vi "benchmark-tagContainer.vi"() -> (3 "write":dbl[](array[numeric])=[4.609181880950928e-05, 2.400779724121094e-06, 7.494449615478516e-07, 2.3156785964965823e-05, 0.00027759432792663576] caption="average" format="%#_6p")   [LabVIEW 2017]
uses:
  c133460f-0aec-4b14-aa01-684956f011bf.vi
  679e9543-87f0-4a91-8f0b-568c5a8b50fd.vi
  TagDB/_Support/DataAccess/_NameCacher.vi
  TagDB/_Support/DataAccess/_datatypeChecker.vi
  TagDB/_Support/DataAccess/TagDB Ref to DVR.vi
  <vilib>/Utility/Data Type/Get Type Information.vi
  <vilib>/Utility/error.llb/Trim Whitespace.vi
  TagDB/_Support/Error/_[error50000]Invalid DB REF.vi
  TagDB/_Support/Error/_[error50002]Invalid DataType.vi
  TagDB/TagDB(DEV).lvlib
panel:
  out "error out":errorcluster
  in  "group name in (Untitled)":string="add more data to containerprivate data"
  out "length":i32=1170
  out "unit (ms)":cluster{dbl[]}[](graph)=[{[4.501104354858398e-05, 5.501508712768555e-05, 6.0143470764160154e-05, 4.501104354858398e-05, 4.500865936279297e-05, 4.001379013061524e-05, 4.5013427734375e-05, 4.000663757324219e-05, 4.500865936279297e-05, 4.5013427734375e-05, 4.5013427734375e-05, 4.5006275177001956e-05, 4.500865936279297e-05, 6.0017108917236326e-05, 4.5123100280761717e-05, 4.500865936279297e-05, 4.500865936279297e-05, 4.5015811920166016e-05, 4.5013427734375e-05, 4.5015811920166016e-05, 4.501104354858398e-05, 4.500865936279297e-05, 5.010128021240234e-05, 4.500865936279297e-05, 4.501104354858398e-05, 4.5013427734375e-05, 4.5006275177001956e-05, 4.500865936279297e-05, 4.501104354858398e-05, 4.502296447753906e-05, 4.5013427734375e-05, 4.500865936279297e-05, 4.501104354858398e-05, 4.501104354858398e-05, 4.5013427734375e-05, 5.0008296966552734e-05, 6.501436233520508e-05, 4.5013427734375e-05, 4.5006275177001956e-05, 4.5013427734375e-05, 4.500865936279297e-05, 4.501104354858398e-05, 5.001068115234375e-05, 4.5013427734375e-05, 4.500865936279297e-05, 4.501104354858398e-05, 4.500865936279297e-05, 4.500865936279297e-05, 4.5013427734375e-05, 4.5013427734375e-05, 4.5006275177001956e-05, 4.500865936279297e-05, 5.001544952392578e-05, 4.500865936279297e-05, 4.501104354858398e-05, 5.501508712768555e-05, 4.5015811920166016e-05, 4.500865936279297e-05, 4.253387451171875e-05, 4.501104354858398e-05, 4.500865936279297e-05, 4.500865936279297e-05, 4.501104354858398e-05, 4.5003890991210935e-05, 4.502058029174805e-05, 4.5015811920166016e-05, 4.5003890991210935e-05, 4.5013427734375e-05, 4.501104354858398e-05, 4.7619342803955076e-05, 4.753589630126953e-05, 4.501104354858398e-05, 4.500865936279297e-05, 5.254030227661133e-05, 4.500865936279297e-05, 4.5006275177001956e-05, 4.5013427734375e-05, 4.500865936279297e-05, 5.000591278076172e-05, 5.001544952392578e-05, 5.003213882446289e-05, 4.5015811920166016e-05, 4.5013427734375e-05, 4.501104354858398e-05, 4.5015811920166016e-05, 4.500865936279297e-05, 4.500865936279297e-05, 4.500865936279297e-05, 4.500865936279297e-05, 4.500865936279297e-05, 4.500865936279297e-05, 4.501104354858398e-05, 4.500865936279297e-05, 4.502296447753906e-05, 4.7540664672851564e-05, 4.501104354858398e-05, 4.5013427734375e-05, 4.501104354858398e-05, 4.500865936279297e-05, 4.500865936279297e-05]}, {[0.0, 0.0, 0.0, 4.999637603759765e-06, 0.0, 4.999637603759765e-06, 4.999637603759765e-06, 5.0044059753417965e-06, 0.0, 4.999637603759765e-06, 0.0, 5.002021789550781e-06, 4.999637603759765e-06, 0.0, 0.0, 0.0, 4.999637603759765e-06, 5.002021789550781e-06, 5.002021789550781e-06, 0.0, 5.002021789550781e-06, 5.0044059753417965e-06, 0.0, 0.0, 0.0, 0.0, 0.0, 4.999637603759765e-06, 4.999637603759765e-06, 5.0044059753417965e-06, 0.0, 0.0, 5.002021789550781e-06, 0.0, 0.0, 0.0, 0.0, 5.002021789550781e-06, 5.0044059753417965e-06, 4.999637603759765e-06, 0.0, 0.0, 0.0, 5.002021789550781e-06, 0.0, 5.002021789550781e-06, 5.0091743469238285e-06, 0.0, 0.0, 4.999637603759765e-06, 4.999637603759765e-06, 4.999637603759765e-06, 0.0, 5.0044059753417965e-06, 5.0044059753417965e-06, 4.999637603759765e-06, 4.99725341796875e-06, 5.002021789550781e-06, 5.0044059753417965e-06, 0.0, 5.0044059753417965e-06, 0.0, 4.999637603759765e-06, 0.0, 0.0, 0.0, 0.0, 0.0, 4.999637603759765e-06, 0.0, 0.0, 4.999637603759765e-06, 5.0044059753417965e-06, 5.0044059753417965e-06, 4.999637603759765e-06, 0.0, 4.999637603759765e-06, 0.0, 0.0, 0.0, 0.0, 0.0, 0.0, 0.0, 4.99725341796875e-06, 0.0, 0.0, 5.002021789550781e-06, 0.0, 5.0067901611328125e-06, 0.0, 5.0044059753417965e-06, 5.0044059753417965e-06, 5.002021789550781e-06, 0.0, 4.999637603759765e-06, 4.999637603759765e-06, 0.0, 4.999637603759765e-06, 0.0]}, {[4.999637603759765e-06, 0.0, 4.963874816894531e-06, 0.0, 0.0, 0.0, 0.0, 0.0, 0.0, 0.0, 4.999637603759765e-06, 0.0, 0.0, 0.0, 4.9686431884765625e-06, 0.0, 0.0, 0.0, 0.0, 4.994869232177734e-06, 0.0, 0.0, 0.0, 0.0, 0.0, 5.0044059753417965e-06, 5.0044059753417965e-06, 0.0, 0.0, 0.0, 0.0, 0.0, 0.0, 0.0, 0.0, 0.0, 0.0, 0.0, 0.0, 0.0, 5.0044059753417965e-06, 0.0, 0.0, 0.0, 0.0, 0.0, 0.0, 0.0, 0.0, 0.0, 0.0, 0.0, 0.0, 0.0, 0.0, 0.0, 0.0, 0.0, 0.0, 0.0, 0.0, 4.999637603759765e-06, 0.0, 0.0, 0.0, 0.0, 0.0, 4.999637603759765e-06, 0.0, 0.0, 0.0, 0.0, 0.0, 0.0, 0.0, 0.0, 0.0, 0.0, 0.0, 0.0, 0.0, 4.99725341796875e-06, 0.0, 0.0, 0.0, 4.999637603759765e-06, 5.0044059753417965e-06, 0.0, 5.0044059753417965e-06, 0.0, 0.0, 0.0, 0.0, 0.0, 0.0, 0.0, 0.0, 4.999637603759765e-06, 0.0, 0.0]}, {[0.0, 4.999637603759765e-06, 0.0, 0.0, 5.0044059753417965e-06, 5.0044059753417965e-06, 4.999637603759765e-06, 5.0044059753417965e-06, 5.002021789550781e-06, 5.0044059753417965e-06, 4.999637603759765e-06, 4.999637603759765e-06, 5.0044059753417965e-06, 9.99927520751953e-06, 5.0044059753417965e-06, 1.0008811950683593e-05, 1.0004043579101563e-05, 1.0004043579101563e-05, 1.0004043579101563e-05, 5.002021789550781e-06, 1.0004043579101563e-05, 9.99927520751953e-06, 1.5003681182861328e-05, 1.5003681182861328e-05, 1.5001296997070313e-05, 9.9945068359375e-06, 9.99927520751953e-06, 9.99927520751953e-06, 1.0001659393310548e-05, 1.4998912811279296e-05, 1.4998912811279296e-05, 1.5003681182861328e-05, 1.5003681182861328e-05, 1.5003681182861328e-05, 2.0003318786621095e-05, 1.500844955444336e-05, 2.000570297241211e-05, 1.5020370483398438e-05, 1.4996528625488281e-05, 2.0003318786621095e-05, 1.4998912811279296e-05, 2.0008087158203125e-05, 2.0003318786621095e-05, 2.0000934600830078e-05, 2.0003318786621095e-05, 2.0008087158203125e-05, 1.999855041503906e-05, 2.0008087158203125e-05, 2.500295639038086e-05, 2.500772476196289e-05, 2.5010108947753908e-05, 2.500772476196289e-05, 2.5005340576171874e-05, 2.5019645690917968e-05, 2.5000572204589844e-05, 2.500772476196289e-05, 2.500295639038086e-05, 2.5005340576171874e-05, 2.5005340576171874e-05, 3.0007362365722656e-05, 2.500295639038086e-05, 2.5019645690917968e-05, 3.0009746551513673e-05, 3.0009746551513673e-05, 3.0007362365722656e-05, 3.000020980834961e-05, 3.0007362365722656e-05, 3.0007362365722656e-05, 3.000497817993164e-05, 3.000497817993164e-05, 3.500938415527344e-05, 3.000497817993164e-05, 3.0007362365722656e-05, 3.5006999969482425e-05, 3.5016536712646485e-05, 4.001379013061524e-05, 3.501176834106445e-05, 3.5006999969482425e-05, 3.500938415527344e-05, 3.500938415527344e-05, 4.000663757324219e-05, 3.5006999969482425e-05, 4.0018558502197264e-05, 4.001140594482422e-05, 4.000663757324219e-05, 3.500938415527344e-05, 3.5006999969482425e-05, 4.00853157043457e-05, 4.000663757324219e-05, 4.0001869201660157e-05, 4.5013427734375e-05, 4.000663757324219e-05, 4.501104354858398e-05, 4.501104354858398e-05, 4.5013427734375e-05, 4.500865936279297e-05, 4.50277328491211e-05, 4.0009021759033204e-05, 4.502296447753906e-05, 4.500865936279297e-05]}, {[4.99725341796875e-06, 1.5001296997070313e-05, 1.5001296997070313e-05, 2.500772476196289e-05, 3.0014514923095703e-05, 3.0002593994140626e-05, 4.0009021759033204e-05, 7.001161575317382e-05, 5.0008296966552734e-05, 5.501031875610351e-05, 6.0017108917236326e-05, 6.501436233520508e-05, 9.001970291137695e-05, 7.501602172851562e-05, 8.501529693603515e-05, 8.502721786499023e-05, 9.001493453979492e-05, 9.501457214355468e-05, 0.00010502099990844727, 0.00011002302169799805, 0.00011460304260253906, 0.00012002706527709961, 0.00012503862380981446, 0.00013002872467041016, 0.00013503074645996094, 0.00014003753662109375, 0.00014503717422485353, 0.00015503644943237304, 0.00015503644943237304, 0.00016003608703613281, 0.00017004013061523439, 0.00017503976821899413, 0.0001806044578552246, 0.00019005537033081054, 0.00019505500793457031, 0.000200045108795166, 0.000200042724609375, 0.0002050495147705078, 0.00021507501602172852, 0.00021257638931274414, 0.0002850651741027832, 0.000225064754486084, 0.00023006439208984376, 0.0002350640296936035, 0.00025005578994750975, 0.00025007009506225583, 0.0002551603317260742, 0.0002612662315368652, 0.0002650594711303711, 0.0002700614929199219, 0.00031507015228271484, 0.0002850604057312012, 0.0002850627899169922, 0.00029006481170654294, 0.0003100800514221191, 0.00030506372451782226, 0.0003050851821899414, 0.0003100967407226563, 0.00032007217407226563, 0.0003250718116760254, 0.00033008813858032227, 0.0003400731086730957, 0.00034508228302001956, 0.00036509513854980467, 0.000355076789855957, 0.00035508394241333006, 0.000360107421875, 0.0003650808334350586, 0.0003751087188720703, 0.000380094051361084, 0.0003900885581970215, 0.0003901028633117676, 0.0004000997543334961, 0.000400092601776123, 0.00040830373764038085, 0.000417630672454834, 0.00041509151458740234, 0.0004601216316223145, 0.00046011924743652346, 0.00043509244918823244, 0.00044509649276733396, 0.00045510292053222654, 0.00046511411666870115, 0.00047010421752929687, 0.0004651880264282227, 0.0004701137542724609, 0.0004752612113952637, 0.0004801154136657715, 0.00048010826110839844, 0.0004943060874938965, 0.0004851078987121582, 0.0004952120780944825, 0.0005151128768920898, 0.0005301427841186523, 0.0005151152610778809, 0.0005151271820068359, 0.0005251169204711914, 0.00053358793258667, 0.0005626559257507324, 0.0005377078056335449]}]
  out "outside":i32=99
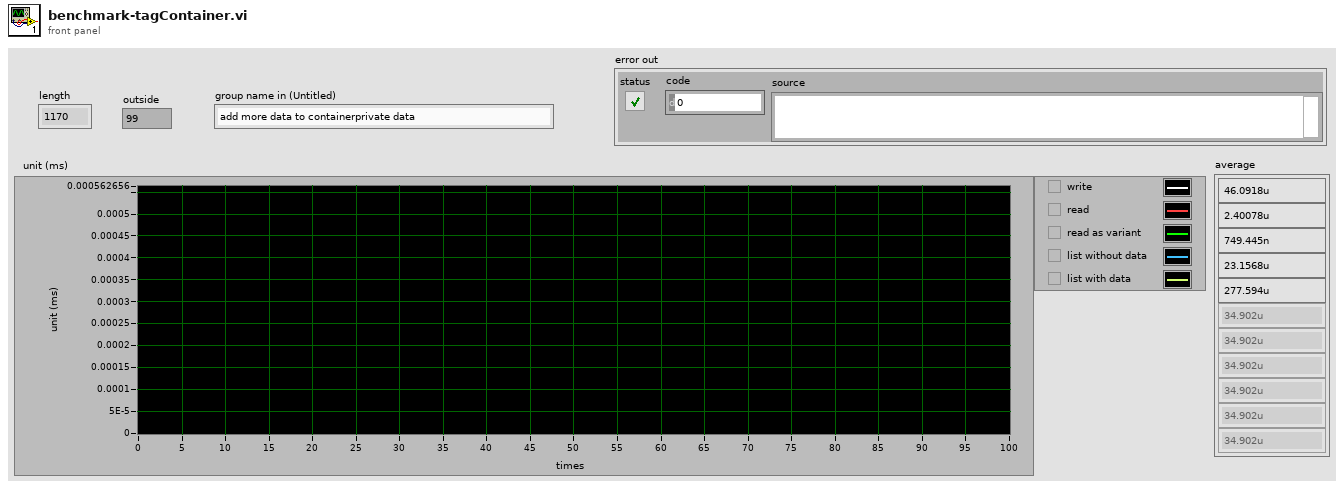
[diagram p1: front panel]
types:
  T1 = enum16{"open", "open or create", "create or replace", "create", "open (read-only)"}
  T2 = cluster{"error constant":errorcluster, "error constant 2":errorcluster, "error constant 3":errorcluster, "error constant 4":errorcluster, "error constant 5":errorcluster, "error constant 6":errorcluster, "error constant 7":errorcluster, "error constant 8":errorcluster, "error constant 9":errorcluster, "error constant 10":errorcluster, "error constant 11":errorcluster, "error constant 12":errorcluster, "error constant 13":errorcluster, "error constant 14":errorcluster, "error constant 15":errorcluster, "error constant 16":errorcluster, "error constant 17":errorcluster, "error constant 18":errorcluster, "error constant 19":errorcluster, "error constant 20":errorcluster, "error constant 21":errorcluster, "error constant 22":errorcluster, "error constant 23":errorcluster, "error constant 24":errorcluster, "error constant 25":errorcluster, "error constant 26":errorcluster, "error constant 27":errorcluster, "error constant 28":errorcluster, "error constant 29":errorcluster, "error constant 30":errorcluster, "error constant 31":errorcluster, "error constant 32":errorcluster, "error constant 33":errorcluster, "error constant 34":errorcluster, "error constant 35":errorcluster, "error constant 36":errorcluster, "error constant 37":errorcluster, "error constant 38":errorcluster, "error constant 39":errorcluster, "error constant 40":errorcluster, "error constant 41":errorcluster, "error constant 42":errorcluster, "error constant 43":errorcluster, "error constant 44":errorcluster, "error constant 45":errorcluster, "error constant 46":errorcluster, "error constant 47":errorcluster, "error constant 48":errorcluster, "error constant 49":errorcluster, "error constant 50":errorcluster, "error constant 51":errorcluster, "error constant 52":errorcluster, "error constant 53":errorcluster, "error constant 54":errorcluster, "error constant 55":errorcluster, "error constant 56":errorcluster, "error constant 57":errorcluster, "error constant 58":errorcluster, "error constant 59":errorcluster, "error constant 60":errorcluster, "error constant 61":errorcluster, "error constant 62":errorcluster, "error constant 63":errorcluster, "error constant 64":errorcluster, "error constant 65":errorcluster, cluster{"error constant":errorcluster, "error constant 2":errorcluster, "error constant 3":errorcluster, "error constant 4":errorcluster, "error constant 5":errorcluster, "error constant 6":errorcluster, "error constant 7":errorcluster, "error constant 8":errorcluster, "error constant 9":errorcluster, "error constant 10":errorcluster, "error constant 11":errorcluster, "error constant 12":errorcluster, "error constant 13":errorcluster, "error constant 14":errorcluster, "error constant 15":errorcluster, "error constant 16":errorcluster, "error constant 17":errorcluster, "error constant 18":errorcluster, "error constant 19":errorcluster, "error constant 20":errorcluster, "error constant 21":errorcluster, "error constant 22":errorcluster, "error constant 23":errorcluster, "error constant 24":errorcluster, "error constant 25":errorcluster, "error constant 26":errorcluster, "error constant 27":errorcluster, "error constant 28":errorcluster, "error constant 29":errorcluster, "error constant 30":errorcluster, "error constant 31":errorcluster, "error constant 32":errorcluster, "error constant 33":errorcluster, "error constant 34":errorcluster, "error constant 35":errorcluster, "error constant 36":errorcluster, "error constant 37":errorcluster, "error constant 38":errorcluster, "error constant 39":errorcluster, "error constant 40":errorcluster, "error constant 41":errorcluster, "error constant 42":errorcluster, "error constant 43":errorcluster, "error constant 44":errorcluster, "error constant 45":errorcluster, "error constant 46":errorcluster, "error constant 47":errorcluster, "error constant 48":errorcluster, "error constant 49":errorcluster, "error constant 50":errorcluster, "error constant 51":errorcluster, "error constant 52":errorcluster, "error constant 53":errorcluster, "error constant 54":errorcluster, "error constant 55":errorcluster, "error constant 56":errorcluster, "error constant 57":errorcluster, "error constant 58":errorcluster, "error constant 59":errorcluster, "error constant 60":errorcluster, "error constant 61":errorcluster, "error constant 62":errorcluster, "error constant 63":errorcluster, "error constant 64":errorcluster, "error constant 65":errorcluster}}
  T3 = typedef "TagDB(DEV).lvlib/TagContainer.ctl" = refnum<k1>
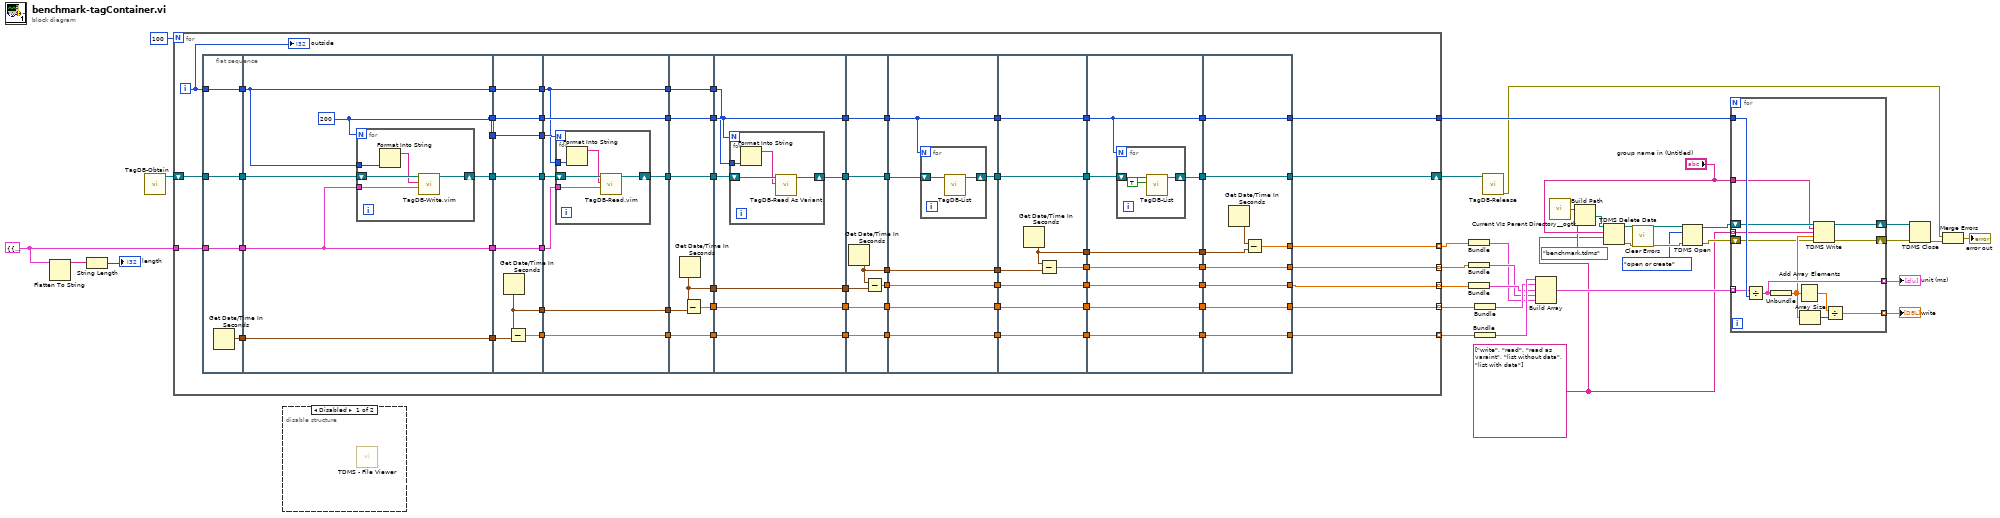
[diagram p0: block diagram]
diagram:
  w1 = string[] ["write", "read", "read as varaint", "list without data", "list with data"]
  w32 = T2 {"error constant"={"status"=FALSE, "code"=0, "source"=""}, "error constant 2"={"status"=FALSE, "code"=0, "source"=""}, "error constant 3"={"status"=FALSE, "code"=0, "source"=""}, "error constant 4"={"status"=FALSE, "code"=0, "source"=""}, "error constant 5"={"status"=FALSE, "code"=0, "source"=""}, "error constant 6"={"status"=FALSE, "code"=0, "source"=""}, "error constant 7"={"status"=FALSE, "code"=0, "source"=""}, "error constant 8"={"status"=FALSE, "code"=0, "source"=""}, "error constant 9"={"status"=FALSE, "code"=0, "source"=""}, "error constant 10"={"status"=FALSE, "code"=0, "source"=""}, "error constant 11"={"status"=FALSE, "code"=0, "source"=""}, "error constant 12"={"status"=FALSE, "code"=0, "source"=""}, "error constant 13"={"status"=FALSE, "code"=0, "source"=""}, "error constant 14"={"status"=FALSE, "code"=0, "source"=""}, "error constant 15"={"status"=FALSE, "code"=0, "source"=""}, "error constant 16"={"status"=FALSE, "code"=0, "source"=""}, "error constant 17"={"status"=FALSE, "code"=0, "source"=""}, "error constant 18"={"status"=FALSE, "code"=0, "source"=""}, "error constant 19"={"status"=FALSE, "code"=0, "source"=""}, "error constant 20"={"status"=FALSE, "code"=0, "source"=""}, "error constant 21"={"status"=FALSE, "code"=0, "source"=""}, "error constant 22"={"status"=FALSE, "code"=0, "source"=""}, "error constant 23"={"status"=FALSE, "code"=0, "source"=""}, "error constant 24"={"status"=FALSE, "code"=0, "source"=""}, "error constant 25"={"status"=FALSE, "code"=0, "source"=""}, "error constant 26"={"status"=FALSE, "code"=0, "source"=""}, "error constant 27"={"status"=FALSE, "code"=0, "source"=""}, "error constant 28"={"status"=FALSE, "code"=0, "source"=""}, "error constant 29"={"status"=FALSE, "code"=0, "source"=""}, "error constant 30"={"status"=FALSE, "code"=0, "source"=""}, "error constant 31"={"status"=FALSE, "code"=0, "source"=""}, "error constant 32"={"status"=FALSE, "code"=0, "source"=""}, "error constant 33"={"status"=FALSE, "code"=0, "source"=""}, "error constant 34"={"status"=FALSE, "code"=0, "source"=""}, "error constant 35"={"status"=FALSE, "code"=0, "source"=""}, "error constant 36"={"status"=FALSE, "code"=0, "source"=""}, "error constant 37"={"status"=FALSE, "code"=0, "source"=""}, "error constant 38"={"status"=FALSE, "code"=0, "source"=""}, "error constant 39"={"status"=FALSE, "code"=0, "source"=""}, "error constant 40"={"status"=FALSE, "code"=0, "source"=""}, "error constant 41"={"status"=FALSE, "code"=0, "source"=""}, "error constant 42"={"status"=FALSE, "code"=0, "source"=""}, "error constant 43"={"status"=FALSE, "code"=0, "source"=""}, "error constant 44"={"status"=FALSE, "code"=0, "source"=""}, "error constant 45"={"status"=FALSE, "code"=0, "source"=""}, "error constant 46"={"status"=FALSE, "code"=0, "source"=""}, "error constant 47"={"status"=FALSE, "code"=0, "source"=""}, "error constant 48"={"status"=FALSE, "code"=0, "source"=""}, "error constant 49"={"status"=FALSE, "code"=0, "source"=""}, "error constant 50"={"status"=FALSE, "code"=0, "source"=""}, "error constant 51"={"status"=FALSE, "code"=0, "source"=""}, "error constant 52"={"status"=FALSE, "code"=0, "source"=""}, "error constant 53"={"status"=FALSE, "code"=0, "source"=""}, "error constant 54"={"status"=FALSE, "code"=0, "source"=""}, "error constant 55"={"status"=FALSE, "code"=0, "source"=""}, "error constant 56"={"status"=FALSE, "code"=0, "source"=""}, "error constant 57"={"status"=FALSE, "code"=0, "source"=""}, "error constant 58"={"status"=FALSE, "code"=0, "source"=""}, "error constant 59"={"status"=FALSE, "code"=0, "source"=""}, "error constant 60"={"status"=FALSE, "code"=0, "source"=""}, "error constant 61"={"status"=FALSE, "code"=0, "source"=""}, "error constant 62"={"status"=FALSE, "code"=0, "source"=""}, "error constant 63"={"status"=FALSE, "code"=0, "source"=""}, "error constant 64"={"status"=FALSE, "code"=0, "source"=""}, "error constant 65"={"status"=FALSE, "code"=0, "source"=""}, {"error constant"={"status"=FALSE, "code"=0, "source"=""}, "error constant 2"={"status"=FALSE, "code"=0, "source"=""}, "error constant 3"={"status"=FALSE, "code"=0, "source"=""}, "error constant 4"={"status"=FALSE, "code"=0, "source"=""}, "error constant 5"={"status"=FALSE, "code"=0, "source"=""}, "error constant 6"={"status"=FALSE, "code"=0, "source"=""}, "error constant 7"={"status"=FALSE, "code"=0, "source"=""}, "error constant 8"={"status"=FALSE, "code"=0, "source"=""}, "error constant 9"={"status"=FALSE, "code"=0, "source"=""}, "error constant 10"={"status"=FALSE, "code"=0, "source"=""}, "error constant 11"={"status"=FALSE, "code"=0, "source"=""}, "error constant 12"={"status"=FALSE, "code"=0, "source"=""}, "error constant 13"={"status"=FALSE, "code"=0, "source"=""}, "error constant 14"={"status"=FALSE, "code"=0, "source"=""}, "error constant 15"={"status"=FALSE, "code"=0, "source"=""}, "error constant 16"={"status"=FALSE, "code"=0, "source"=""}, "error constant 17"={"status"=FALSE, "code"=0, "source"=""}, "error constant 18"={"status"=FALSE, "code"=0, "source"=""}, "error constant 19"={"status"=FALSE, "code"=0, "source"=""}, "error constant 20"={"status"=FALSE, "code"=0, "source"=""}, "error constant 21"={"status"=FALSE, "code"=0, "source"=""}, "error constant 22"={"status"=FALSE, "code"=0, "source"=""}, "error constant 23"={"status"=FALSE, "code"=0, "source"=""}, "error constant 24"={"status"=FALSE, "code"=0, "source"=""}, "error constant 25"={"status"=FALSE, "code"=0, "source"=""}, "error constant 26"={"status"=FALSE, "code"=0, "source"=""}, "error constant 27"={"status"=FALSE, "code"=0, "source"=""}, "error constant 28"={"status"=FALSE, "code"=0, "source"=""}, "error constant 29"={"status"=FALSE, "code"=0, "source"=""}, "error constant 30"={"status"=FALSE, "code"=0, "source"=""}, "error constant 31"={"status"=FALSE, "code"=0, "source"=""}, "error constant 32"={"status"=FALSE, "code"=0, "source"=""}, "error constant 33"={"status"=FALSE, "code"=0, "source"=""}, "error constant 34"={"status"=FALSE, "code"=0, "source"=""}, "error constant 35"={"status"=FALSE, "code"=0, "source"=""}, "error constant 36"={"status"=FALSE, "code"=0, "source"=""}, "error constant 37"={"status"=FALSE, "code"=0, "source"=""}, "error constant 38"={"status"=FALSE, "code"=0, "source"=""}, "error constant 39"={"status"=FALSE, "code"=0, "source"=""}, "error constant 40"={"status"=FALSE, "code"=0, "source"=""}, "error constant 41"={"status"=FALSE, "code"=0, "source"=""}, "error constant 42"={"status"=FALSE, "code"=0, "source"=""}, "error constant 43"={"status"=FALSE, "code"=0, "source"=""}, "error constant 44"={"status"=FALSE, "code"=0, "source"=""}, "error constant 45"={"status"=FALSE, "code"=0, "source"=""}, "error constant 46"={"status"=FALSE, "code"=0, "source"=""}, "error constant 47"={"status"=FALSE, "code"=0, "source"=""}, "error constant 48"={"status"=FALSE, "code"=0, "source"=""}, "error constant 49"={"status"=FALSE, "code"=0, "source"=""}, "error constant 50"={"status"=FALSE, "code"=0, "source"=""}, "error constant 51"={"status"=FALSE, "code"=0, "source"=""}, "error constant 52"={"status"=FALSE, "code"=0, "source"=""}, "error constant 53"={"status"=FALSE, "code"=0, "source"=""}, "error constant 54"={"status"=FALSE, "code"=0, "source"=""}, "error constant 55"={"status"=FALSE, "code"=0, "source"=""}, "error constant 56"={"status"=FALSE, "code"=0, "source"=""}, "error constant 57"={"status"=FALSE, "code"=0, "source"=""}, "error constant 58"={"status"=FALSE, "code"=0, "source"=""}, "error constant 59"={"status"=FALSE, "code"=0, "source"=""}, "error constant 60"={"status"=FALSE, "code"=0, "source"=""}, "error constant 61"={"status"=FALSE, "code"=0, "source"=""}, "error constant 62"={"status"=FALSE, "code"=0, "source"=""}, "error constant 63"={"status"=FALSE, "code"=0, "source"=""}, "error constant 64"={"status"=FALSE, "code"=0, "source"=""}, "error constant 65"={"status"=FALSE, "code"=0, "source"=""}}}
  n1 = Flatten To String(anything=w32) -> (data string=w31:string)  [unwired: 3 in, 2 out]
  n2 = String Length(string=w31) -> (length=→"length":i32)
  n3 = call "TagDB-Obtain.vi"() -> ("TagContainer"=w34:T3)  [unwired: 5 in, 2 out]
  n4 = for {
    N: 100 -> [_]
    tunnel: [w103] -> w26 mode=indexing
    tunnel: [w102] -> w28
    tunnel: w32 -> [w92]
    shift-right: [w90] -> w33
    shift-left: w34 -> [w91]
    tunnel: [w85] -> w27 mode=indexing
    tunnel: [w72] -> w24 mode=indexing
    tunnel: [w38] -> w23 mode=indexing
    tunnel: [w37] -> w22 mode=indexing
    i -> [w100]
    n5 = flat-sequence {
      tunnel: [w109] -> w105
      tunnel: [w108] -> w95
      tunnel: [w107] -> w94
      tunnel: [w106] -> w93
      tunnel: w91 -> [w108]
      tunnel: w92 -> [w107]
      tunnel: w100 -> [w106]
      tunnel: w105 -> [w115]
      tunnel: [w115] -> w104
      tunnel: [w111] -> w101
      tunnel: [w113] -> w96
      tunnel: w95 -> [w114]
      tunnel: w94 -> [w110]
      tunnel: w93 -> [w112]
      tunnel: [w111] -> w83
      tunnel: [w112] -> w80
      tunnel: [w110] -> w78
      tunnel: w104 -> [w125]
      tunnel: w101 -> [w127]
      tunnel: [w128] -> w99
      tunnel: [w127] -> w98
      tunnel: [w126] -> w97
      tunnel: w96 -> [w126]
      tunnel: [w121] -> w87
      tunnel: w83 -> [w124]
      tunnel: [w124] -> w82
      tunnel: [w123] -> w81
      tunnel: w80 -> [w123]
      tunnel: [w122] -> w79
      tunnel: w78 -> [w122]
      tunnel: w99 -> [w136]
      tunnel: w98 -> [w135]
      tunnel: w97 -> [w133]
      tunnel: [w136] -> w89
      tunnel: [w135] -> w88
      tunnel: w87 -> [w134]
      tunnel: [w134] -> w86
      tunnel: [w132] -> w84
      tunnel: w82 -> [w131]
      tunnel: w81 -> [w129]
      tunnel: w79 -> [w130]
      tunnel: [w129] -> w71
      tunnel: w89 -> [w148]
      tunnel: w88 -> [w145]
      tunnel: w86 -> [w147]
      tunnel: w84 -> [w143]
      tunnel: [w148] -> w70
      tunnel: [w145] -> w69
      tunnel: [w146] -> w68
      tunnel: [w144] -> w67
      tunnel: w71 -> [w144]
      tunnel: [w143] -> w66
      tunnel: [w142] -> w65
      tunnel: w70 -> [w155]
      tunnel: w69 -> [w152]
      tunnel: w68 -> [w154]
      tunnel: [w155] -> w77
      tunnel: [w152] -> w76
      tunnel: [w153] -> w75
      tunnel: [w154] -> w74
      tunnel: [w149] -> w73
      tunnel: w67 -> [w151]
      tunnel: w66 -> [w150]
      tunnel: w65 -> [w149]
      tunnel: w77 -> [w166]
      tunnel: w76 -> [w165]
      tunnel: w75 -> [w164]
      tunnel: w74 -> [w163]
      tunnel: w73 -> [w162]
      tunnel: [w166] -> w64
      tunnel: [w165] -> w63
      tunnel: [w164] -> w62
      tunnel: [w163] -> w61
      tunnel: [w161] -> w60
      tunnel: [w160] -> w54
      tunnel: w64 -> [w173]
      tunnel: w63 -> [w167]
      tunnel: w62 -> [w170]
      tunnel: w61 -> [w172]
      tunnel: w60 -> [w171]
      tunnel: [w173] -> w59
      tunnel: [w167] -> w58
      tunnel: [w169] -> w57
      tunnel: [w172] -> w56
      tunnel: [w171] -> w55
      tunnel: w54 -> [w168]
      tunnel: [w168] -> w53
      tunnel: w59 -> [w183]
      tunnel: w58 -> [w182]
      tunnel: w57 -> [w181]
      tunnel: w56 -> [w180]
      tunnel: w55 -> [w179]
      tunnel: w53 -> [w178]
      tunnel: [w183] -> w52
      tunnel: [w182] -> w51
      tunnel: [w181] -> w50
      tunnel: [w180] -> w49
      tunnel: [w179] -> w48
      tunnel: [w177] -> w47
      tunnel: [w176] -> w40
      tunnel: w52 -> [w191]
      tunnel: w51 -> [w184]
      tunnel: w50 -> [w187]
      tunnel: w49 -> [w190]
      tunnel: w48 -> [w189]
      tunnel: w47 -> [w188]
      tunnel: [w191] -> w46
      tunnel: [w184] -> w45
      tunnel: [w186] -> w44
      tunnel: [w190] -> w43
      tunnel: [w189] -> w42
      tunnel: [w188] -> w41
      tunnel: w40 -> [w185]
      tunnel: [w185] -> w39
      tunnel: [w198] -> w37
      tunnel: [w199] -> w72
      tunnel: [w200] -> w85
      tunnel: [w201] -> w90
      tunnel: [w202] -> w102
      tunnel: [w203] -> w103
      tunnel: w46 -> [w203]
      tunnel: w45 -> [w202]
      tunnel: w44 -> [w201]
      tunnel: w43 -> [w200]
      tunnel: w42 -> [w199]
      tunnel: w41 -> [w198]
      tunnel: w39 -> [w196]
      tunnel: [w195] -> w38
      frame #0 {
        n6 = Get Date/Time In Seconds() -> (seconds since 1Jan1904=w109:timestamp)
      }
      frame #1 {
        w111 = 200
        n7 = for {
          N: w111 -> [_]
          tunnel: w110 -> [w118]
          tunnel: w112 -> [w117]
          shift-right: [w119] -> w113
          shift-left: w114 -> [w120]
          n8 = Format Into String(w117) -> (resulting string=w116:string)  [unwired: 3 in, 1 out]
          n9 = call "TagDB-Write.vim"("Value"=w118, "name"=w116, "TagContainer"=w120) -> ("TagContainer(dup)"=w119:T3)  [unwired: 6 in, 2 out]
        }
      }
      frame #2 {
        n10 = Get Date/Time In Seconds() -> (seconds since 1Jan1904=w121:timestamp)
        n11 = Subtract(x=w121, y=w125) -> (x-y=w128:dbl)
      }
      frame #3 {
        n12 = for {
          N: w131 -> [_]
          shift-right: [w140] -> w132
          shift-left: w133 -> [w141]
          tunnel: w129 -> [w138]
          tunnel: w130 -> [w137]
          n13 = Format Into String(w138) -> (resulting string=w139:string)  [unwired: 3 in, 1 out]
          n14 = call "TagDB-Read.vim"("Type"=w137, "name"=w139, "TagContainer"=w141) -> ("TagContainer(dup)"=w140:T3)  [unwired: 3 in, 5 out]
        }
      }
      frame #4 {
        n15 = Get Date/Time In Seconds() -> (seconds since 1Jan1904=w142:timestamp)
        n16 = Subtract(x=w142, y=w147) -> (x-y=w146:dbl)
      }
      frame #5 {
        n17 = for {
          N: w152 -> [_]
          shift-right: [w158] -> w153
          shift-left: w150 -> [w159]
          tunnel: w151 -> [w156]
          n18 = Format Into String(w156) -> (resulting string=w157:string)  [unwired: 3 in, 1 out]
          n19 = call "TagDB-Read As Variant.vi"("name"=w157, "TagContainer"=w159) -> ("TagContainer(dup)"=w158:T3)  [unwired: 4 in, 5 out]
        }
      }
      frame #6 {
        n20 = Get Date/Time In Seconds() -> (seconds since 1Jan1904=w160:timestamp)
        n21 = Subtract(x=w160, y=w162) -> (x-y=w161:dbl)
      }
      frame #7 {
        n22 = for {
          N: w167 -> [_]
          shift-right: [w174] -> w169
          shift-left: w170 -> [w175]
          n23 = call "TagDB-List.vi"("TagContainer"=w175) -> ("TagContainer(dup)"=w174:T3)  [unwired: 7 in, 3 out]
        }
      }
      frame #8 {
        n24 = Get Date/Time In Seconds() -> (seconds since 1Jan1904=w176:timestamp)
        n25 = Subtract(x=w176, y=w178) -> (x-y=w177:dbl)
      }
      frame #9 {
        n26 = for {
          N: w184 -> [_]
          shift-right: [w193] -> w186
          shift-left: w187 -> [w194]
          n27 = call "TagDB-List.vi"("with Data?(F)"=TRUE, "TagContainer"=w194) -> ("TagContainer(dup)"=w193:T3)  [unwired: 6 in, 3 out]
        }
      }
      frame #10 {
        n28 = Get Date/Time In Seconds() -> (seconds since 1Jan1904=w197:timestamp)
        n29 = Subtract(x=w197, y=w196) -> (x-y=w195:dbl)
      }
    }
    "outside" <- w100
  }
  n30 = disable-structure shown="Disabled" {
    frame Disabled {
      n31 = call <vilib>:"TDMS - File Viewer.vi"() -> ()  [unwired: 6 in, 2 out]
    }
    frame Enabled {
    }
  }
  n32 = Bundle(w23) -> (w17:cluster{dbl[]})  [unwired: 1 in]
  n33 = Bundle(w22) -> (w18:cluster{dbl[]})  [unwired: 1 in]
  n34 = Bundle(w24) -> (w19:cluster{dbl[]})  [unwired: 1 in]
  n35 = Bundle(w27) -> (w20:cluster{dbl[]})  [unwired: 1 in]
  n36 = Bundle(w26) -> (w21:cluster{dbl[]})  [unwired: 1 in]
  n37 = call "TagDB-Release.vi"("TagContainer"=w33) -> ("error out"=w3:errorcluster)  [unwired: 10 in]
  n38 = Build Array(w21, w20, w19, w18, w17) -> (w25:cluster{dbl[]}[])
  n39 = call <userlib>:"Current VIs Parent Directory__ogtk.vi"() -> ("Parent Directory (+ Relative)"=w9:path)  [unwired: 5 in]
  n40 = Build Path(base path=w9, name or relative path="benchmark.tdms") -> (appended path=w8:path)
  n41 = TDMS Delete Data(9:w1, 10:"group name in (Untitled)", 11:w8) -> (0:w11:errorcluster, 3:w10:path)  [unwired: 4 in]
  n42 = call <vilib>:"Clear Errors.vi"("error in (no error)"=w11) -> ("error out"=w6:errorcluster)  [unwired: 5 in, 1 out]
  n43 = TDMS Open(8:w6, 10:T1."open or create" ("operation (0:open)"), 11:w10) -> (0:w14:errorcluster, 3:w13:refnum<k34>)  [unwired: 4 in]
  n44 = for {
    tunnel: [w216] -> w30 mode=indexing
    tunnel: [w211] -> w29 mode=indexing
    tunnel: w28 -> [w213]
    tunnel: w25 -> [w212] mode=indexing
    shift-right: [w209] -> w16
    shift-left: w13 -> [w208]
    shift-right: [w207] -> w15
    shift-left: w14 -> [w206]
    tunnel: w1 -> [w205] mode=indexing
    tunnel: "group name in (Untitled)" -> [w204]
    n45 = Divide(x=w212, y=w213) -> (x/y=w211:cluster{dbl[]})
    n46 = Unbundle(w211) -> (w210:dbl[])
    n47 = Add Array Elements(numeric array=w210) -> (sum=w215:dbl)
    n48 = Array Size(array=w210) -> (size(s)=w214:i32)
    n49 = TDMS Write(0:w208, 5:w204, 7:w205, 9:w210, 11:w206) -> (4:w209:refnum<k34>, 15:w207:errorcluster)  [unwired: 1 in, 2 out]
    n50 = Divide(x=w215, y=w214) -> (x/y=w216:dbl)
  }
  "unit (ms)" <- w29
  "write" <- w30
  n51 = TDMS Close(8:w15, 11:w16) -> (0:w4:errorcluster)  [unwired: 1 out]
  n52 = Merge Errors(w3, w4) -> (→"error out":errorcluster)
